vi "getValueFromXMLNative.vi"(8 "error in (no error)":errorcluster, 10 "eventXML":refnum<k20>, 11 "RfRamp in":refnum<class "RfRamp.lvclass">) -> (0 "error out":errorcluster, 2 "eventXML out":refnum<k20>, 3 "RfRamp out":refnum<class "RfRamp.lvclass">)   [LabVIEW 2011, in "Tools.lvlib" / "Scripting.lvlib" / "RfRamp.lvclass"]
uses:
  RfRamp.lvclass
  RfRamp.lvclass/RfRamp.ctl
  <vilib>/xml/Close Reference(Node).vi
  <vilib>/xml/NI_XML.lvlib
  ScriptEvent.lvclass
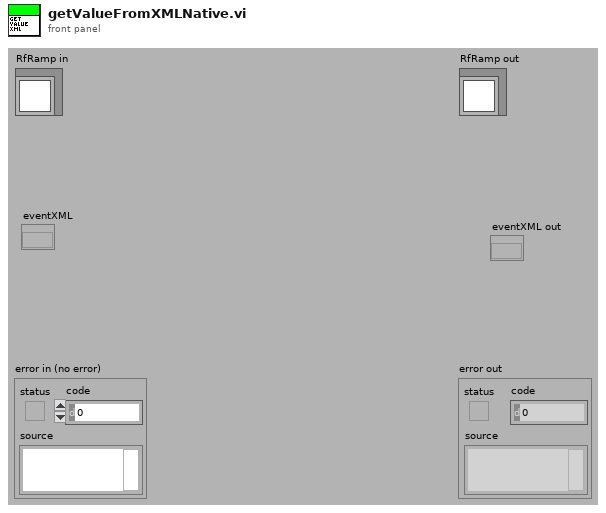
[diagram p1: front panel]
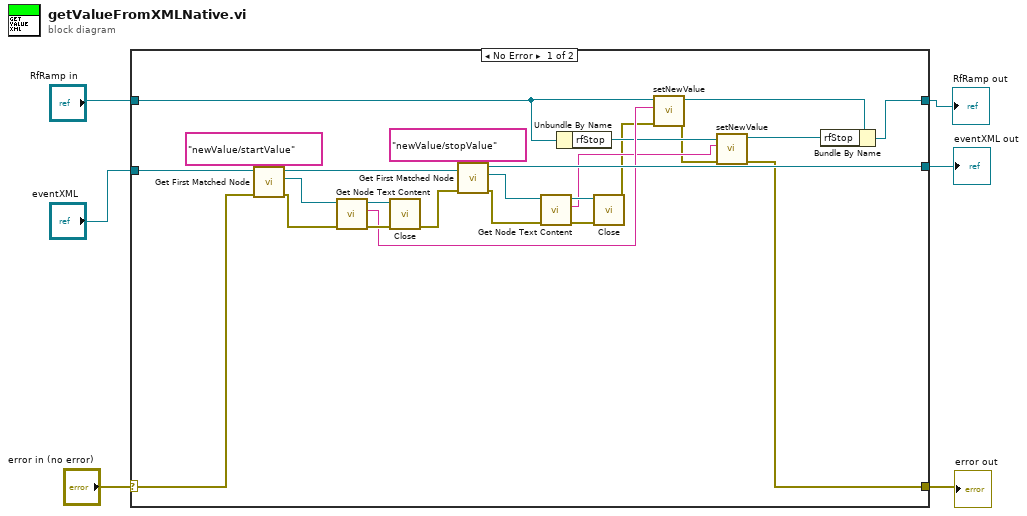
[diagram p0: block diagram]
diagram:
  n1 = case shown="No Error" "error in (no error)" {
    selector: "error in (no error)" -> [w28 w33]
    tunnel: [w10 w33] -> w2
    tunnel: [w7 w34] -> w3
    tunnel: "RfRamp in" -> [w16 w34]
    tunnel: "eventXML" -> [w29 w32]
    tunnel: [w17 w32] -> w1
    frame No Error {
      n2 = call <vilib>:"Get First Matched Node.vi"("error in (no error)"=w28, "XPath expression"="newValue/startValue", "node in"=w29) -> ("error out"=w25:errorcluster, "node result"=w26:refnum<k20>, "node out"=w19:refnum<k20>)  [unwired: 6 in]
      n3 = call <vilib>:"Get Node Text Content.vi"("error in (no error)"=w25, "node in"=w26) -> ("error out"=w30:errorcluster, "node text"=w15:string, "node out"=w31:refnum<k20>)  [unwired: 7 in]
      n4 = call-poly <vilib>:"Close.vi"("error in (no error)"=w30, "node"=w31) -> ("error out"=w18:errorcluster)  [unwired: 7 in]
      n5 = call <vilib>:"Get First Matched Node.vi"("error in (no error)"=w18, "XPath expression"="newValue/stopValue", "node in"=w19) -> ("error out"=w24:errorcluster, "node result"=w23:refnum<k20>, "node out"=w17:refnum<k20>)  [unwired: 6 in]
      n6 = call <vilib>:"Get Node Text Content.vi"("error in (no error)"=w24, "node in"=w23) -> ("error out"=w21:errorcluster, "node text"=w13:string, "node out"=w20:refnum<k20>)  [unwired: 7 in]
      n7 = Unbundle By Name(w16) -> ("rfStop"=w14:refnum<class "rf.lvclass">)
      n8 = call-poly <vilib>:"Close.vi"("error in (no error)"=w21, "node"=w20) -> ("error out"=w11:errorcluster)  [unwired: 7 in]
      n9 = call "setNewValue.vi"("error in (no error)"=w11, "newValue"=w15, "ScriptEvent.lvclass in"=w16) -> ("error out"=w12:errorcluster, "ScriptEvent.lvclass out"=w9:refnum<class "RfRamp.lvclass">)  [unwired: 7 in]
      n10 = call "setNewValue.vi"("error in (no error)"=w12, "newValue"=w13, "ScriptEvent.lvclass in"=w14) -> ("error out"=w10:errorcluster, "ScriptEvent.lvclass out"=w8:refnum<class "rf.lvclass">)  [unwired: 7 in]
      n11 = Bundle By Name(cluster=w9, "rfStop"=w8) -> (w7:refnum<class "RfRamp.lvclass">)
    }
    frame Error {
    }
  }
  "error out" <- w2
  "RfRamp out" <- w3
  "eventXML out" <- w1
